vi "Read.vi"(8 "error in (no error)":errorcluster, 11 "Subset_STR in":refnum<class "Subset_STR.lvclass">) -> (0 "error out":errorcluster, 2 "String":string, 3 "Subset_STR out":refnum<class "Subset_STR.lvclass">)   [LabVIEW 2021, in "Subset_STR.lvclass"]
uses:
  Subset_STR.lvclass
  Subset_STR.lvclass/Subset_STR.ctl
  Abs_Types/String/Abs_String.lvclass
  Abs_Types/Numeric/Abs_Numeric.lvclass
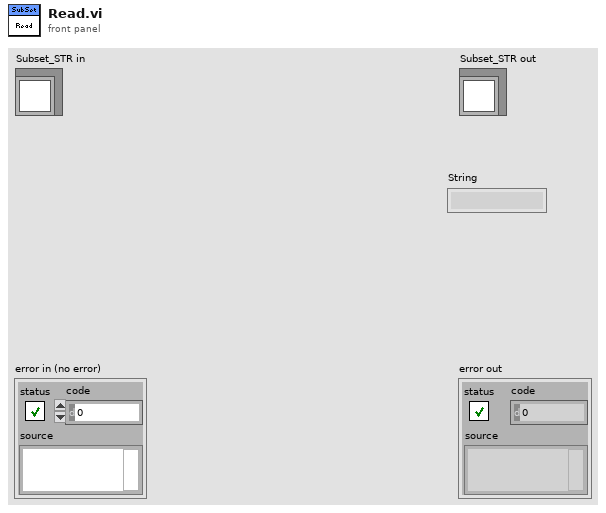
[diagram p1: front panel]
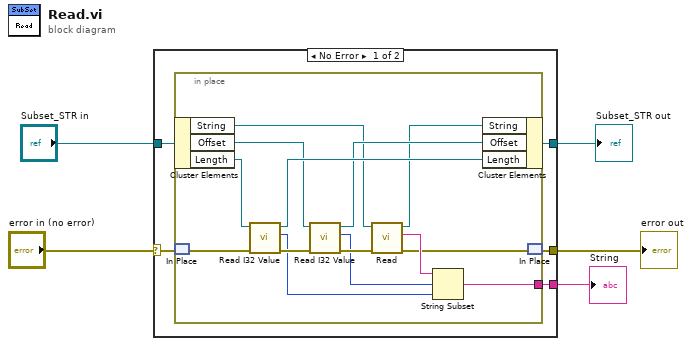
[diagram p0: block diagram]
diagram:
  n1 = case shown="No Error" "error in (no error)" {
    selector: "error in (no error)" -> [w9 w25]
    tunnel: "Subset_STR in" -> [w10 w26]
    tunnel: [w8 _] -> w3
    tunnel: [w7 w25] -> w2
    tunnel: [w6 w26] -> w1
    frame No Error {
      n2 = in-place {
        in-place-border: [w20] -> w8
        n3 = in-place-cluster #1(w10) -> ("String"=w12:refnum<class "Abs_String.lvclass">, "Offset"=w14:refnum<class "Abs_Numeric.lvclass">, "Length"=w16:refnum<class "Abs_Numeric.lvclass">)
        n4 = in-place-match #2(w9) -> (w23:errorcluster)
        n5 = call-dynamic "Read I32 Value.vi"("error in (no error)"=w23, "Numeric in"=w16) -> ("error out"=w24:errorcluster, "I32"=w17:i32, "Numeric out"=w15:refnum<class "Abs_Numeric.lvclass">)  [unwired: 7 in]
        n6 = call-dynamic "Read I32 Value.vi"("error in (no error)"=w24, "Numeric in"=w14) -> ("error out"=w22:errorcluster, "I32"=w19:i32, "Numeric out"=w13:refnum<class "Abs_Numeric.lvclass">)  [unwired: 7 in]
        n7 = call-dynamic "Read.vi"("error in (no error)"=w22, "Abs_String in"=w12) -> ("error out"=w18:errorcluster, "String"=w21:string, "Abs_String out"=w11:refnum<class "Abs_String.lvclass">)  [unwired: 7 in]
        n8 = String Subset(string=w21, offset (0)=w19, length (rest)=w17) -> (substring=w20:string)
        n9 = in-place-cluster #1("String"=w11, "Offset"=w13, "Length"=w15) -> (w6:refnum<class "Subset_STR.lvclass">)
        n10 = in-place-match #2(w18) -> (w7:errorcluster)
      }
    }
    frame Error {
    }
  }
  "error out" <- w2
  "Subset_STR out" <- w1
  "String" <- w3
